vi "sub step control.vi"(9 "First time?":bool, 10 "Step cluster":T3={"Step number"=0, "Step Name"="", "Step name enum"=enum."Init NI", "Start condition 1 name"="", "Start condition 1 comparator"="", "Start condition 1 value"=0.0, "Start condition 2 name"="", "Start condition 2 comparator"="", "Start condition 2 value"=0.0, "Start condition 3 name"="", "Start condition 3 comparator"="", "Start condition 3 value"=0.0, "End condition 1 name"="", "End condition 1 comparator"="", "End condition 1 value"=0.0, "End condition 2 name"="", "End condition 2 comparator"="", "End condition 2 value"=0.0, "End condition 3 name"="", "End condition 3 comparator"="", "End condition 3 value"=0.0, "Constant condition 1 name"="", "Constant condition 1 comparator"="", "Constant condition 1 value"=0.0, "Constant condition 2 name"="", "Constant condition 2 comparator"="", "Constant condition 2 value"=0.0, "Constant condition 3 name"="", "Constant condition 3 comparator"="", "Constant condition 3 value"=0.0, "Duration, mS"=0.0, "Max Duration, mS"=0.0}, 11 "Sub step":T1) -> (3 "Sub step out":T1)   [LabVIEW 2014]
uses:
  Control/Step name enum.ctl
  Control/Sub step profiler.ctl
  Test status global.vi
  <vilib>/Automated Test Systems Ltd/General Tools/Stopwatch/Stop watch/Stop watch.lvlib
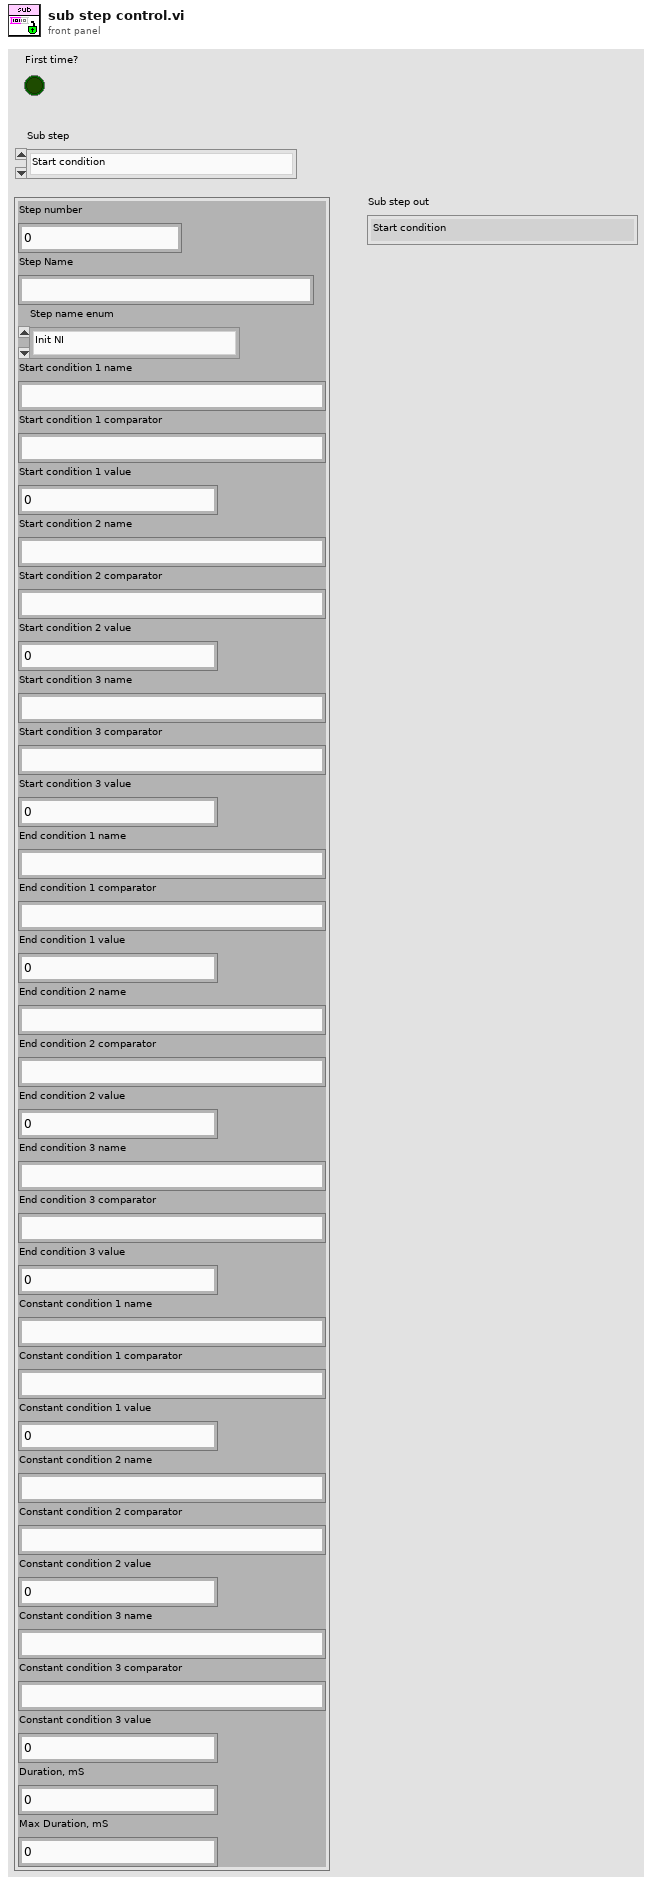
[diagram p1: front panel]
types:
  T1 = typedef "Sub step profiler.ctl" = enum16{"Start condition", "Constant condition", "End condition", "Fail", "Complete"}
  T2 = typedef "Step name enum.ctl" = enum16{"Default", "Idle", "Init Ard", "Init SM", "Init NI", "Run", "Close"}
  T3 = cluster{"Step number":i32, "Step Name":string, "Step name enum":T2, "Start condition 1 name":string, "Start condition 1 comparator":string, "Start condition 1 value":dbl, "Start condition 2 name":string, "Start condition 2 comparator":string, "Start condition 2 value":dbl, "Start condition 3 name":string, "Start condition 3 comparator":string, "Start condition 3 value":dbl, "End condition 1 name":string, "End condition 1 comparator":string, "End condition 1 value":dbl, "End condition 2 name":string, "End condition 2 comparator":string, "End condition 2 value":dbl, "End condition 3 name":string, "End condition 3 comparator":string, "End condition 3 value":dbl, "Constant condition 1 name":string, "Constant condition 1 comparator":string, "Constant condition 1 value":dbl, "Constant condition 2 name":string, "Constant condition 2 comparator":string, "Constant condition 2 value":dbl, "Constant condition 3 name":string, "Constant condition 3 comparator":string, "Constant condition 3 value":dbl, "Duration, mS":dbl, "Max Duration, mS":dbl}
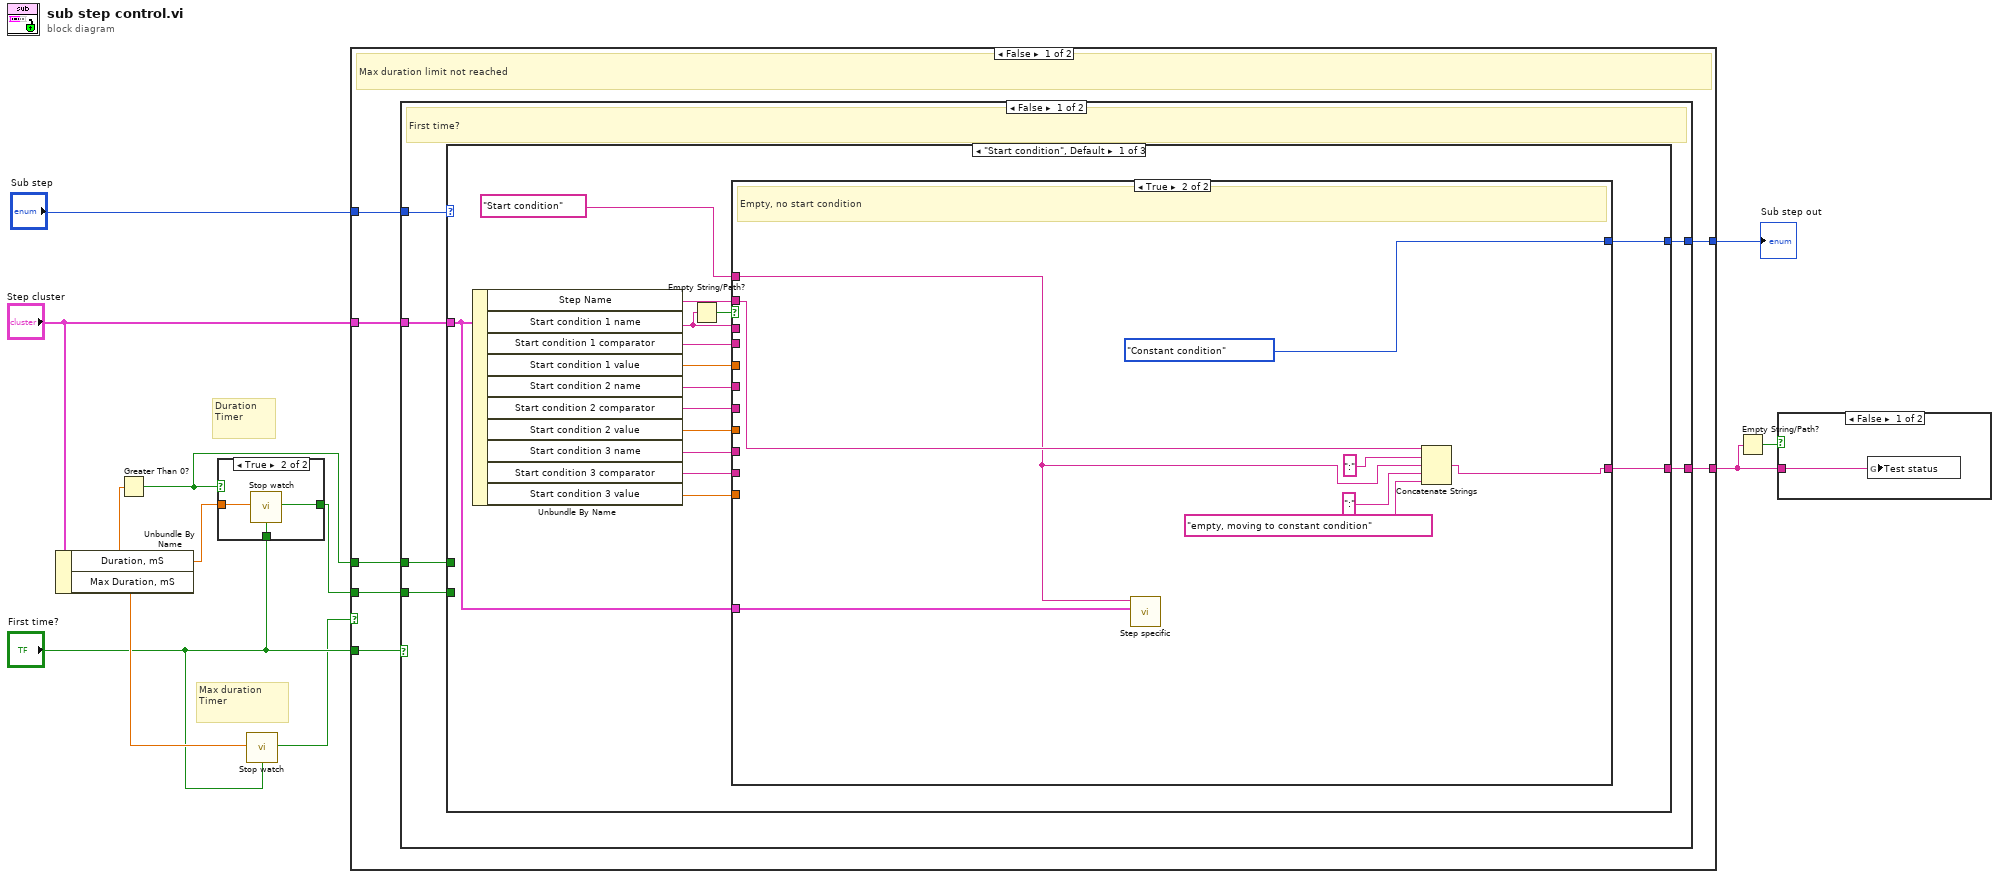
[diagram p0: block diagram]
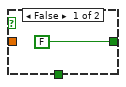
[diagram p3: hidden frame]
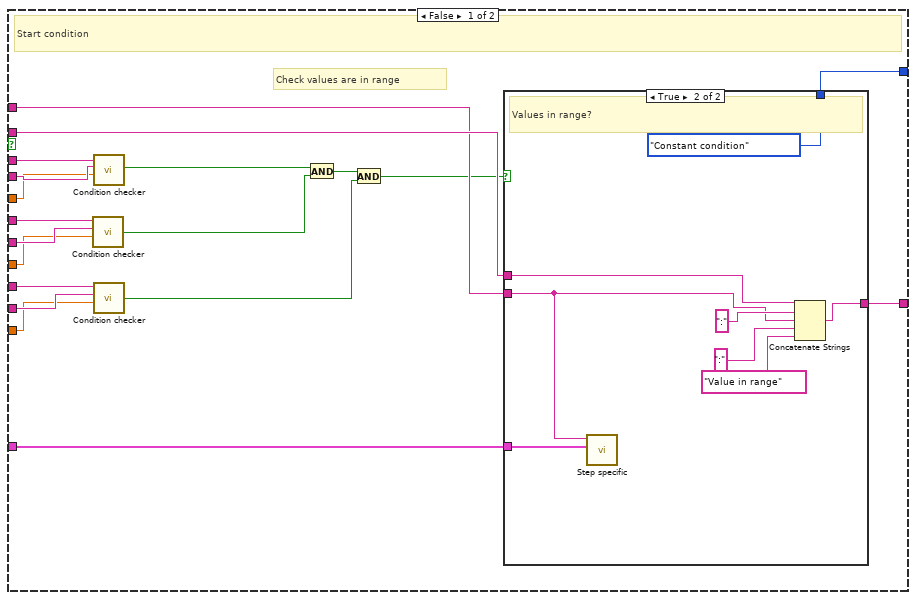
[diagram p4: hidden frame]
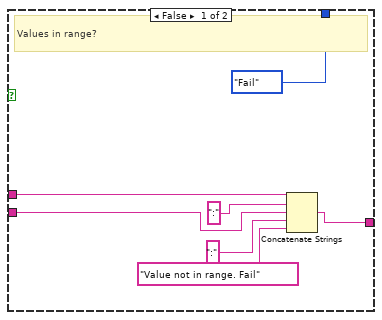
[diagram p5: hidden frame]
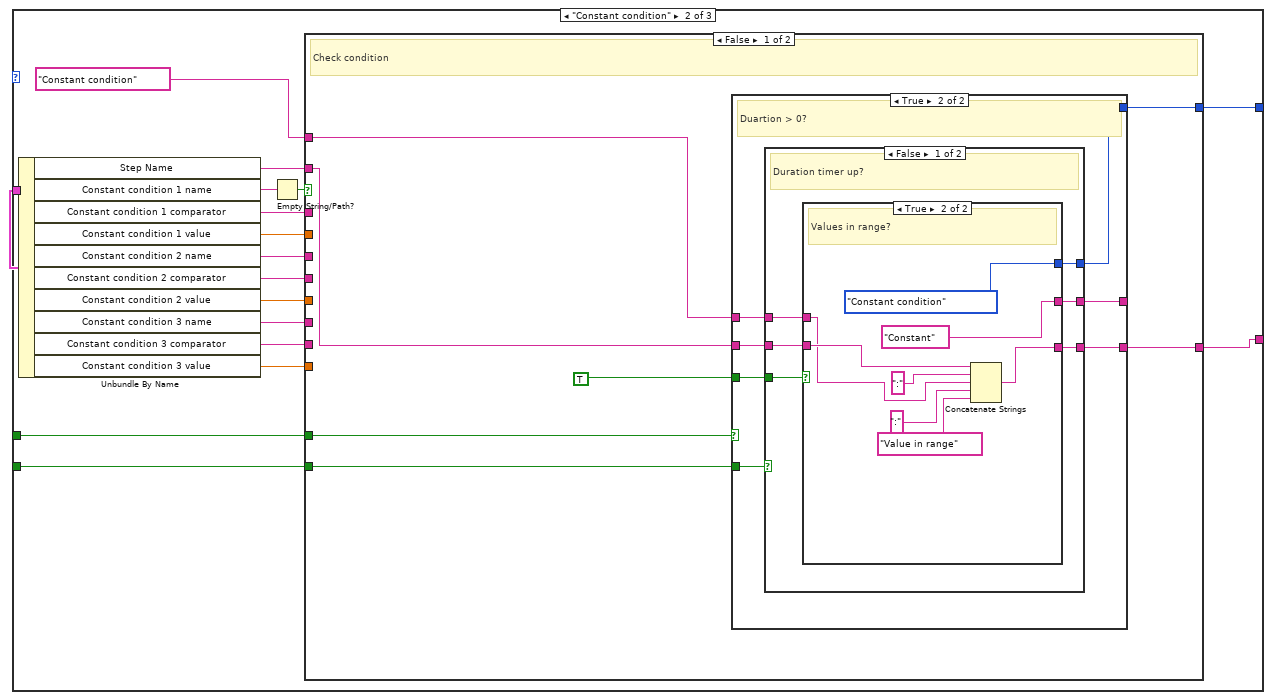
[diagram p6: hidden frame]
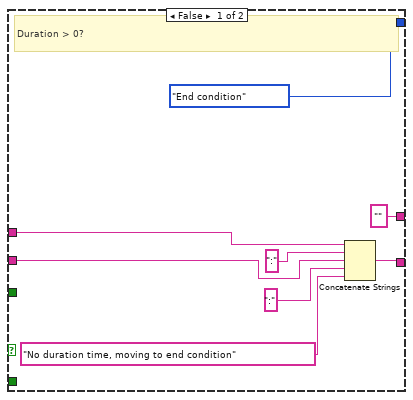
[diagram p7: hidden frame]
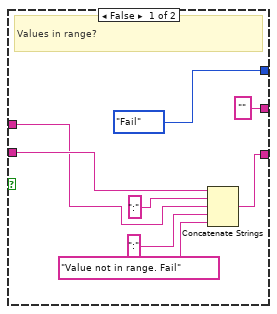
[diagram p8: hidden frame]
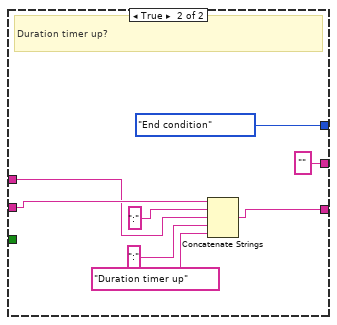
[diagram p9: hidden frame]
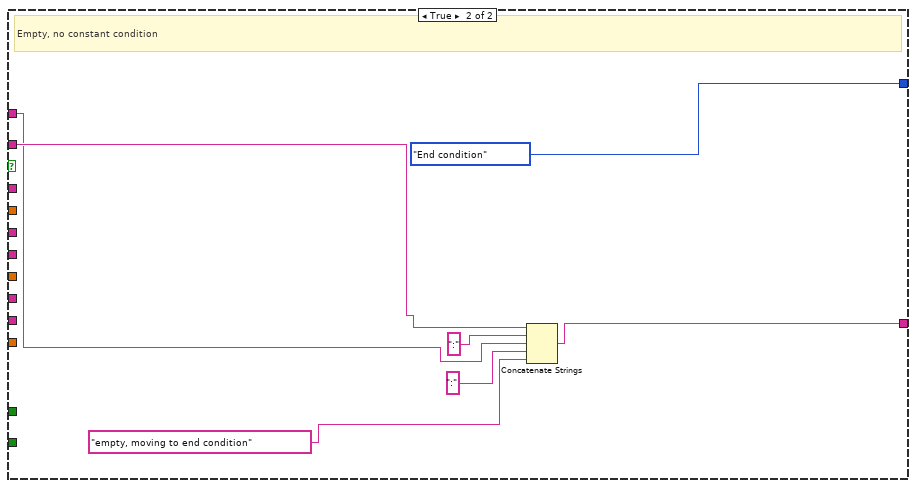
[diagram p10: hidden frame]
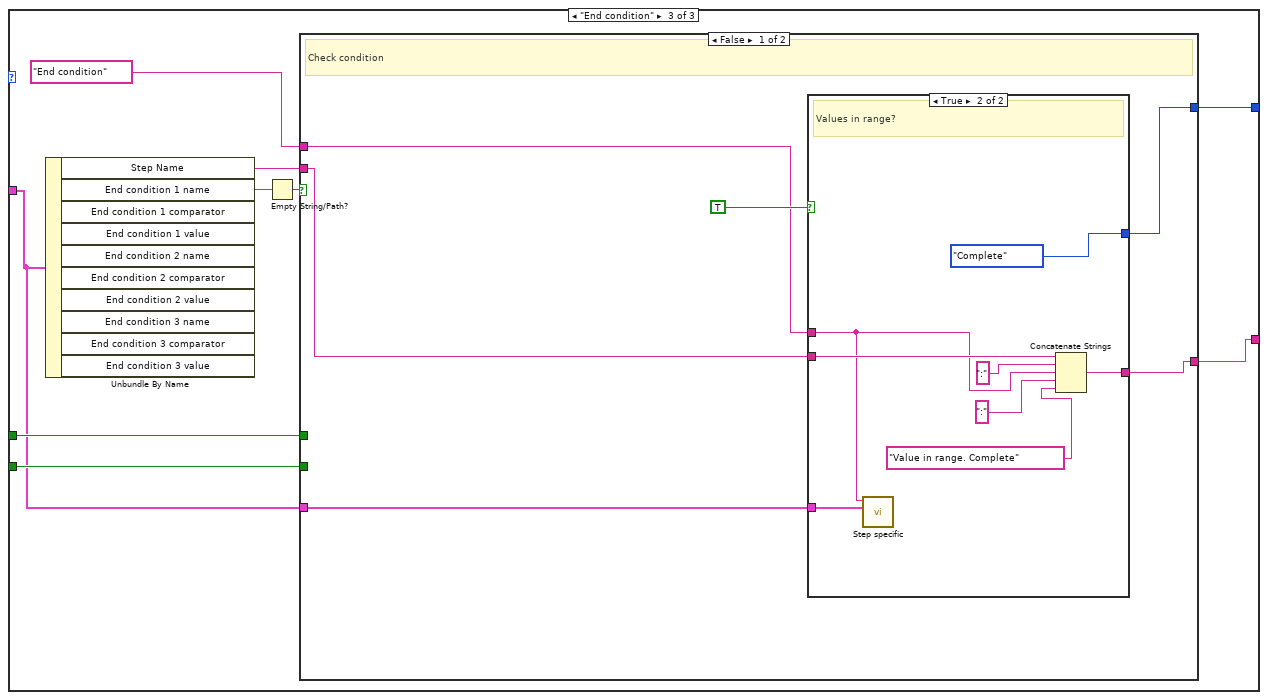
[diagram p11: hidden frame]
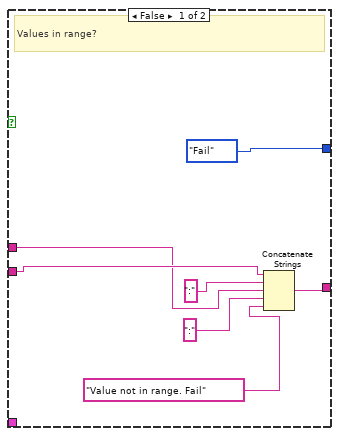
[diagram p12: hidden frame]
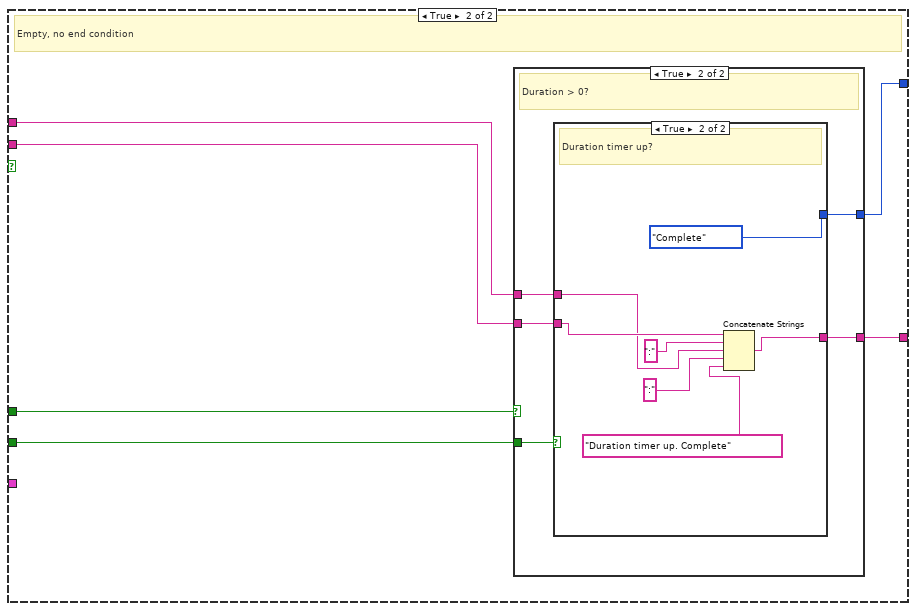
[diagram p13: hidden frame]
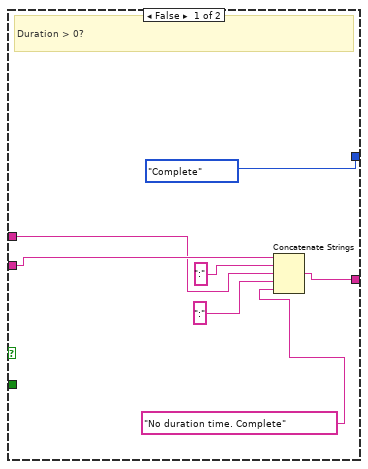
[diagram p14: hidden frame]
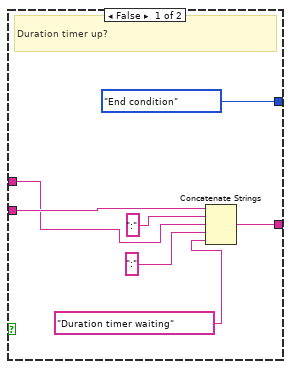
[diagram p15: hidden frame]
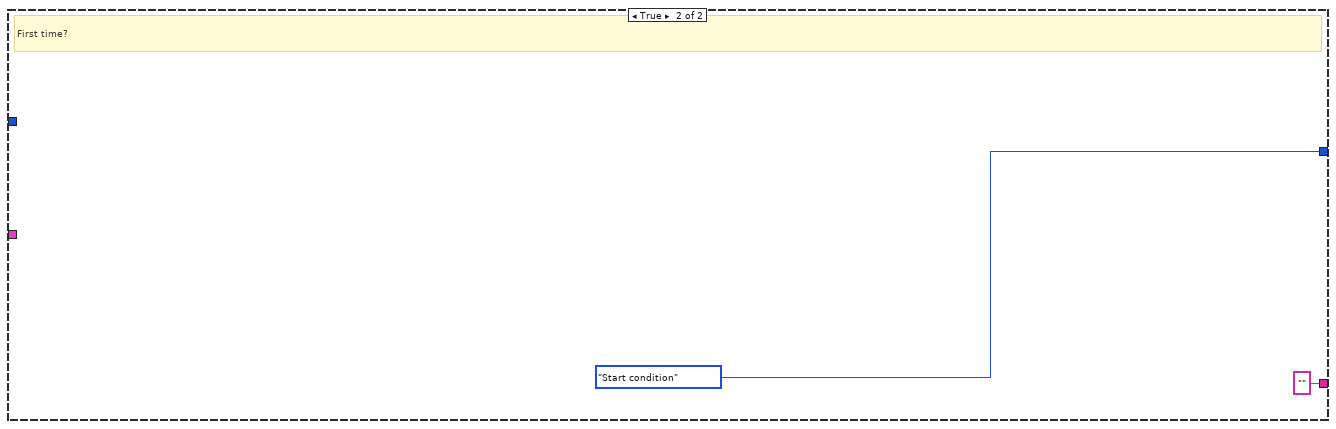
[diagram p16: hidden frame]
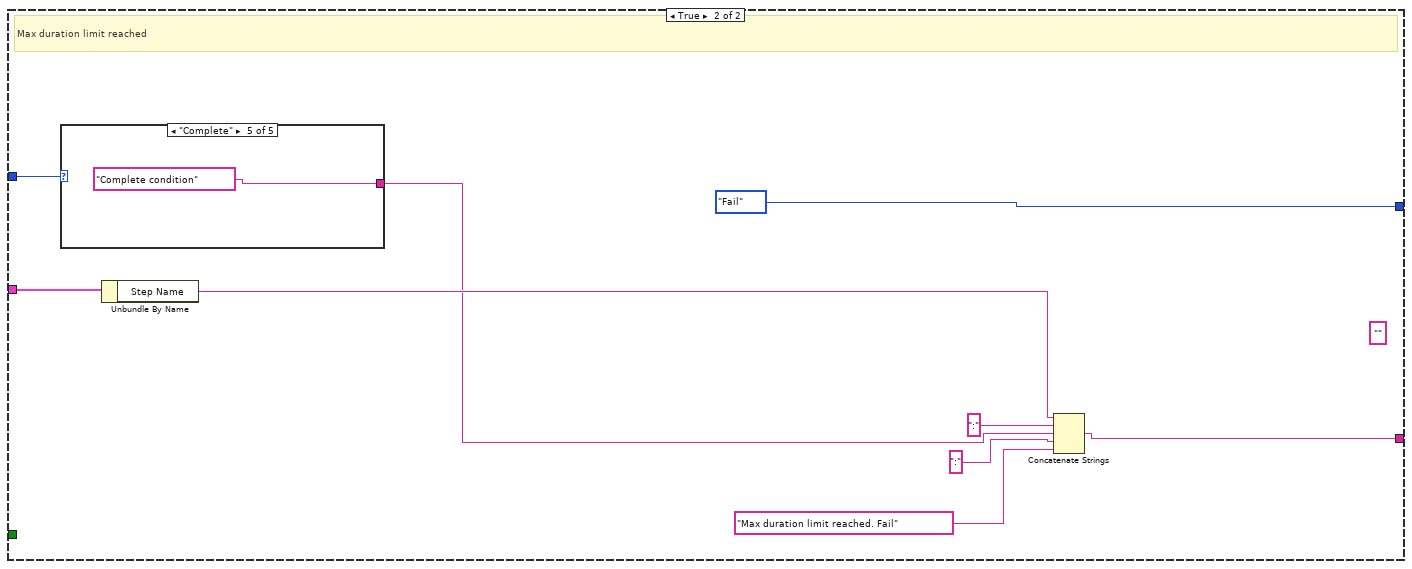
[diagram p17: hidden frame]
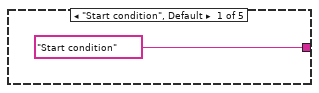
[diagram p18: hidden frame]
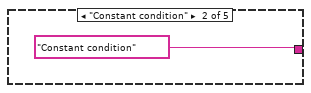
[diagram p19: hidden frame]
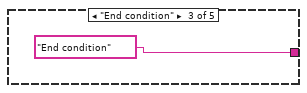
[diagram p20: hidden frame]
diagram:
  # "Duration\nTimer"
  # "Max duration\nTimer"
  n1 = Unbundle By Name("Step cluster") -> ("Duration, mS"=w8:dbl, "Max Duration, mS"=w3:dbl)
  n2 = Greater Than 0?(x=w8) -> (x > 0?=w6:bool)
  n3 = case shown="True" w6 {
    tunnel: "First time?" -> [_ w15]
    tunnel: w8 -> [_ w13]
    tunnel: [FALSE ("Timer up") w14] -> w7
    frame False {
    }
    frame True {
      n4 = call <vilib>:"Stop watch.vi"("Time to wait, mS"=w13, "reset timer"=w15) -> ("Timer up"=w14:bool)  [unwired: 12 in, 1 out]
    }
  }
  n5 = call <vilib>:"Stop watch.vi"("Time to wait, mS"=w3, "reset timer"="First time?") -> ("Timer up"=w1:bool)  [unwired: 12 in, 1 out]
  n6 = case shown="False" w1 {
    tunnel: "Sub step" -> [w22 w232]
    tunnel: [w21 Sub_step_profiler."Fail" ("Sub step")] -> w10
    tunnel: "Step cluster" -> [w20 w233]
    tunnel: "First time?" -> [w19 _]
    tunnel: w7 -> [w18 _]
    tunnel: w6 -> [w17 _]
    tunnel: [w16 w226] -> w5
    frame False {
      # "Max duration limit not reached"
      n7 = case shown="False" w19 {
        tunnel: w22 -> [w28 _]
        tunnel: [w27 Sub_step_profiler."Start condition" ("Sub step")] -> w21
        tunnel: w20 -> [w26 _]
        tunnel: w18 -> [w25 _]
        tunnel: w17 -> [w24 _]
        tunnel: [w23 ""] -> w16
        frame False {
          # "First time?"
          n8 = case shown="\"Start condition\", Default" w28 {
            tunnel: w26 -> [w29 w100 w162]
            tunnel: [w42 w99 w168] -> w27
            tunnel: w25 -> [_ w89 w166]
            tunnel: w24 -> [_ w90 w167]
            tunnel: [w31 w86 w163] -> w23
            frame "Start condition", Default {
              n9 = Unbundle By Name(w29) -> ("Step Name"=w33:string, "Start condition 1 name"=w32:string, "Start condition 1 comparator"=w41:string, "Start condition 1 value"=w37:dbl, "Start condition 2 name"=w38:string, "Start condition 2 comparator"=w40:string, "Start condition 2 value"=w36:dbl, "Start condition 3 name"=w35:string, "Start condition 3 comparator"=w39:string, "Start condition 3 value"=w34:dbl)
              n10 = Empty String/Path?(string/path=w32) -> (empty?=w43:bool)
              n11 = case shown="True" w43 {
                tunnel: [w62 Sub_step_profiler."Constant condition" ("Sub step")] -> w42
                tunnel: w41 -> [w57 _]
                tunnel: w40 -> [w54 _]
                tunnel: w39 -> [w51 _]
                tunnel: w38 -> [w55 _]
                tunnel: w37 -> [w56 _]
                tunnel: w36 -> [w53 _]
                tunnel: w35 -> [w52 _]
                tunnel: w34 -> [w50 _]
                tunnel: w33 -> [w61 w80]
                tunnel: w32 -> [w58 _]
                tunnel: [w60 w81] -> w31
                tunnel: "Start condition" -> [w59 w79]
                tunnel: w29 -> [w44 w78]
                frame False {
                  # "Check values are in range"
                  # "Start condition"
                  n12 = call "Condition checker.vi"("Condition name"=w55, "Condition comparator"=w54, "Condition value"=w53) -> ("Condition in spec?"=w48:bool)  [unwired: 5 in]
                  n13 = call "Condition checker.vi"("Condition name"=w58, "Condition comparator"=w57, "Condition value"=w56) -> ("Condition in spec?"=w49:bool)  [unwired: 5 in]
                  n14 = call "Condition checker.vi"("Condition name"=w52, "Condition comparator"=w51, "Condition value"=w50) -> ("Condition in spec?"=w46:bool)  [unwired: 5 in]
                  n15 = And(x=w49, y=w48) -> (x .and. y?=w47:bool)
                  n16 = And(x=w47, y=w46) -> (x .and. y?=w45:bool)
                  n17 = case shown="True" w45 {
                    tunnel: [Sub_step_profiler."Fail" ("Sub step") Sub_step_profiler."Constant condition" ("Sub step")] -> w62
                    tunnel: w61 -> [w68 w73]
                    tunnel: [w64 w72] -> w60
                    tunnel: w59 -> [w63 w71]
                    tunnel: w44 -> [_ w70]
                    frame False {
                      # "Values in range?"
                      n18 = Concatenate Strings(w68, ":", w63, ":", "Value not in range. Fail" ("string")) -> (w64:string)
                    }
                    frame True {
                      # "Values in range?"
                      n19 = call "Step specific.vi"("Step cluster"=w70, "Task condition"=w71) -> ()  [unwired: 10 in]
                      n20 = Concatenate Strings(w73, ":", w71, ":", "Value in range" ("string")) -> (w72:string)
                    }
                  }
                }
                frame True {
                  # "Empty, no start condition"
                  n21 = call "Step specific.vi"("Step cluster"=w78, "Task condition"=w79) -> ()  [unwired: 10 in]
                  n22 = Concatenate Strings(w80, ":", w79, ":", "empty, moving to constant condition" ("string")) -> (w81:string)
                }
              }
            }
            frame "Constant condition" {
              n23 = Unbundle By Name(w100) -> ("Step Name"=w87:string, "Constant condition 1 name"=w101:string, "Constant condition 1 comparator"=w98:string, "Constant condition 1 value"=w97:dbl, "Constant condition 2 name"=w96:string, "Constant condition 2 comparator"=w95:string, "Constant condition 2 value"=w94:dbl, "Constant condition 3 name"=w93:string, "Constant condition 3 comparator"=w92:string, "Constant condition 3 value"=w91:dbl)
              n24 = Empty String/Path?(string/path=w101) -> (empty?=w102:bool)
              n25 = case shown="False" w102 {
                tunnel: [w109 Sub_step_profiler."End condition" ("Sub step")] -> w99
                tunnel: w98 -> [_ _]
                tunnel: w97 -> [_ _]
                tunnel: w96 -> [_ _]
                tunnel: w95 -> [_ _]
                tunnel: w94 -> [_ _]
                tunnel: w93 -> [_ _]
                tunnel: w92 -> [_ _]
                tunnel: w91 -> [_ _]
                tunnel: w90 -> [w108 _]
                tunnel: w89 -> [w107 _]
                tunnel: "Constant condition" -> [w104 w157]
                tunnel: w87 -> [w105 w158]
                tunnel: [w103 w155] -> w86
                frame False {
                  # "Check condition"
                  n26 = case shown="True" w108 {
                    tunnel: [Sub_step_profiler."End condition" ("Sub step") w124] -> w109
                    tunnel: w107 -> [_ w123]
                    tunnel: TRUE -> [_ w122]
                    tunnel: w105 -> [w111 w121]
                    tunnel: w104 -> [w112 w120]
                    tunnel: [w113 w119] -> w103
                    tunnel: ["" w118] -> _
                    frame False {
                      # "Duration > 0?"
                      n27 = Concatenate Strings(w112, ":", w111, ":", "No duration time, moving to end condition" ("string")) -> (w113:string)
                    }
                    frame True {
                      # "Duartion > 0?"
                      n28 = case shown="False" w123 {
                        tunnel: [w130 Sub_step_profiler."End condition" ("Sub step")] -> w124
                        tunnel: w122 -> [w129 _]
                        tunnel: w121 -> [w128 w149]
                        tunnel: w120 -> [w127 w148]
                        tunnel: [w126 w150] -> w119
                        tunnel: [w125 ""] -> w118
                        frame False {
                          # "Duration timer up?"
                          n29 = case shown="True" w129 {
                            tunnel: [Sub_step_profiler."Fail" ("Sub step") Sub_step_profiler."Constant condition" ("Sub step")] -> w130
                            tunnel: w128 -> [w134 w142]
                            tunnel: w127 -> [w133 w141]
                            tunnel: [w132 w140] -> w126
                            tunnel: ["" "Constant"] -> w125
                            frame False {
                              # "Values in range?"
                              n30 = Concatenate Strings(w134, ":", w133, ":", "Value not in range. Fail" ("string")) -> (w132:string)
                            }
                            frame True {
                              # "Values in range?"
                              n31 = Concatenate Strings(w142, ":", w141, ":", "Value in range" ("string")) -> (w140:string)
                            }
                          }
                        }
                        frame True {
                          # "Duration timer up?"
                          n32 = Concatenate Strings(w149, ":", w148, ":", "Duration timer up" ("string")) -> (w150:string)
                        }
                      }
                    }
                  }
                }
                frame True {
                  # "Empty, no constant condition"
                  n33 = Concatenate Strings(w158, ":", w157, ":", "empty, moving to end condition" ("string")) -> (w155:string)
                }
              }
            }
            frame "End condition" {
              n34 = Unbundle By Name(w162) -> ("Step Name"=w165:string, "End condition 1 name"=w170:string)  [unwired: 8 out]
              n35 = Empty String/Path?(string/path=w170) -> (empty?=w169:bool)
              n36 = case shown="False" w169 {
                tunnel: [w176 w197] -> w168
                tunnel: w167 -> [_ w196]
                tunnel: w166 -> [_ w195]
                tunnel: w165 -> [w173 w193]
                tunnel: "End condition" -> [w172 w192]
                tunnel: [w174 w194] -> w163
                tunnel: w162 -> [w171 _]
                frame False {
                  # "Check condition"
                  n37 = case shown="True" TRUE {
                    tunnel: [Sub_step_profiler."Fail" ("Sub step") Sub_step_profiler."Complete" ("Sub step")] -> w176
                    tunnel: [w180 w188] -> w174
                    tunnel: w173 -> [w179 w187]
                    tunnel: w172 -> [w178 w184]
                    tunnel: w171 -> [_ w185]
                    frame False {
                      # "Values in range?"
                      n38 = Concatenate Strings(w179, ":", w178, ":", "Value not in range. Fail" ("string")) -> (w180:string)
                    }
                    frame True {
                      # "Values in range?"
                      n39 = call "Step specific.vi"("Step cluster"=w185, "Task condition"=w184) -> ()  [unwired: 10 in]
                      n40 = Concatenate Strings(w187, ":", w184, ":", "Value in range. Complete" ("string")) -> (w188:string)
                    }
                  }
                }
                frame True {
                  # "Empty, no end condition"
                  n41 = case shown="True" w196 {
                    tunnel: [Sub_step_profiler."Complete" ("Sub step") w209] -> w197
                    tunnel: w195 -> [_ w208]
                    tunnel: [w198 w207] -> w194
                    tunnel: w193 -> [w200 w206]
                    tunnel: w192 -> [w199 w205]
                    frame False {
                      # "Duration > 0?"
                      n42 = Concatenate Strings(w200, ":", w199, ":", "No duration time. Complete" ("string")) -> (w198:string)
                    }
                    frame True {
                      # "Duration > 0?"
                      n43 = case shown="True" w208 {
                        tunnel: [Sub_step_profiler."End condition" ("Sub step") Sub_step_profiler."Complete" ("Sub step")] -> w209
                        tunnel: [w213 w219] -> w207
                        tunnel: w206 -> [w212 w218]
                        tunnel: w205 -> [w211 w217]
                        frame False {
                          # "Duration timer up?"
                          n44 = Concatenate Strings(w212, ":", w211, ":", "Duration timer waiting" ("string")) -> (w213:string)
                        }
                        frame True {
                          # "Duration timer up?"
                          n45 = Concatenate Strings(w218, ":", w217, ":", "Duration timer up. Complete" ("string")) -> (w219:string)
                        }
                      }
                    }
                  }
                }
              }
            }
          }
        }
        frame True {
          # "First time?"
        }
      }
    }
    frame True {
      (unwired) ""
      # "Max duration limit reached"
      n46 = case shown="\"Complete\"" w232 {
        tunnel: ["Start condition" "Constant condition" "End condition" "Fail condition" "Complete condition"] -> w229
        frame "Start condition", Default {
        }
        frame "Constant condition" {
        }
        frame "End condition" {
        }
        frame "Fail" {
        }
        frame "Complete" {
        }
      }
      n47 = Unbundle By Name(w233) -> ("Step Name"=w231:string)
      n48 = Concatenate Strings(w231, ":" ("string"), w229, ":" ("string"), "Max duration limit reached. Fail" ("string")) -> (w226:string)
    }
  }
  "Sub step out" <- w10
  n49 = Empty String/Path?(string/path=w5) -> (empty?=w4:bool)
  n50 = case shown="False" w4 {
    tunnel: w5 -> [w240 _]
    frame False {
      n51 = global write "Test status global.vi" "Test status"(w240) -> ()
    }
    frame True {
    }
  }
